vi "Print Footprint v8.1 add to 48 cases.vi"() -> ()   [LabVIEW 2018]
panel:
  in  "Manual Input":string
  out "error out 2":errorcluster
  out "error out":errorcluster
  out "Ring Text":string
  in  "Enter time limit":dbl=10.0
  out "Role":i32[][](array[numeric])=[[1, 0], [3, 0], [10, 0], [18, 0]]
  in  "Manual Input":i32[][](array[numeric])=[[1, 0], [3, 0], [5, 0], [7, 0], [12, 0], [13, 0], [17, 0], [20, 1]]
  out "Numeric 4":i32=7
  out "element":i32=6
  out "Match":u16(ring)=18 items=["0", "1", "2"]
  in  "Select Role":u16(ring)=18 items=["Thyroiditis"=48, "Kidney disease"=47, "Prinzmetal angina"=46, "Gallstones"=45, "Appendicitis"=44, "Heart valve problem"=43, "Enlarged heart"=42, "Staff 20"=41, "Doctor 18"=40, "Doctor 17"=39, "Doctor 16"=38, "Doctor 15"=37, "Doctor 14"=36, "Doctor 13"=35, "Doctor 12"=34, "Nurse 11"=33, "Doctor 10"=32, "Staff 9"=31, "Doctor 8"=30, "Nurse 7"=29, "Doctor 6"=28, "Doctor 5"=27, "Doctor 4"=26, "Doctor 3"=25, "Nurse 1"=24, "Manual Input"=0, "Common cold"=1, "Skin rash"=2, "Anemia"=3, "High blood pressure"=4, "Flu"=5, "Laryngitis"=6, "Strep throat"=7, "Sinus disease"=8, "Sprained wrist"=9, "Sprained ankle"=10, "Allergy"=11, "Lung disease"=12, "Intoxication"=13, "Pneumonia"=14, "Tuberculosis"=15, "Fractured nose"=16, "Fractured rib"=17, "Arrhythmia"=18, "Atherosclerosis"=19, "Anxiety"=20, "Insomnia"=21, "Paranoia"=22, "Diarrhea"=23]
  in  "stop":bool
  in  "Start":bool
  out "Syntetic":i32[][](array[numeric])=[[2, 1], [2, 1], [1, 0], [2, 1], [3, 0], [10, 0], [18, 0]]
  in  "Resting Room #":dbl=20.0
  in  "Toilet Room #":dbl=2.0
  in  "Resting limit":dbl
  in  "Toilet limit":dbl=6.0
  in  "Run for":i32=100
  in  "Enter Rnd Lmt":dbl=2.0
  out "offset past number":i32
  out "for time":i32=2
  out "time":dbl=13.0
  out "at nroom":i32=17
  out "Numeric 3":i32=2
  out "x-1":i32=2
  out "Numeric":i32=13
  out "x+y":dbl
  out "x+1":i32=6
  out "path":path=path "C:/Users/synti/OneDrive/Desktop/NI/new/100.png"
  out "Rec Frame":i32=100
  in  "Record?":bool=TRUE
  out "read":picture
  in  "Entering time":dbl
  out "Footprint":picture
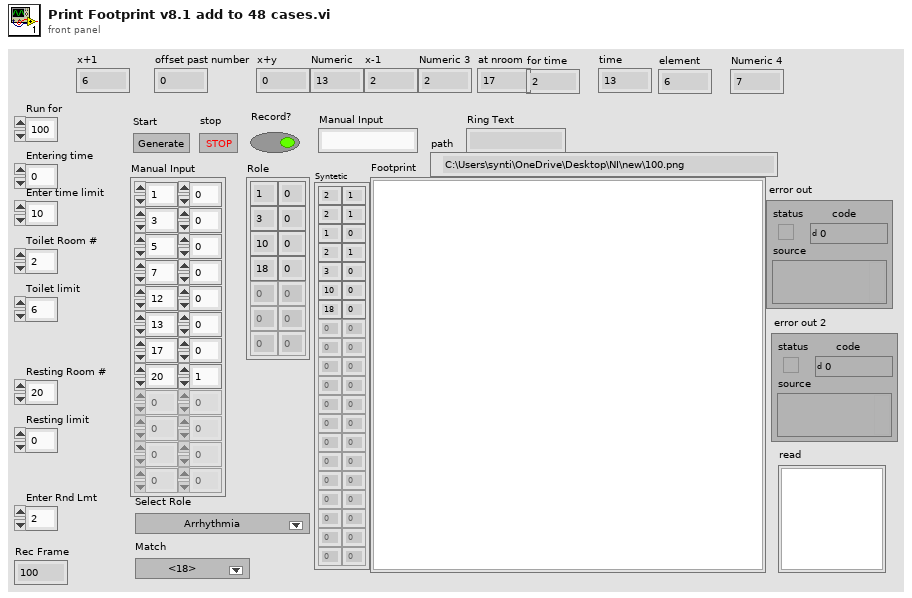
[diagram p1: front panel]
types:
  T1 = typedef "imagedata.ctl" = cluster{"image type":i32, "image depth":i32, "image":u8[], "mask":u8[], "colors":u32[], "Rectangle":cluster{"left":i16, "top":i16, "right":i16, "bottom":i16}}
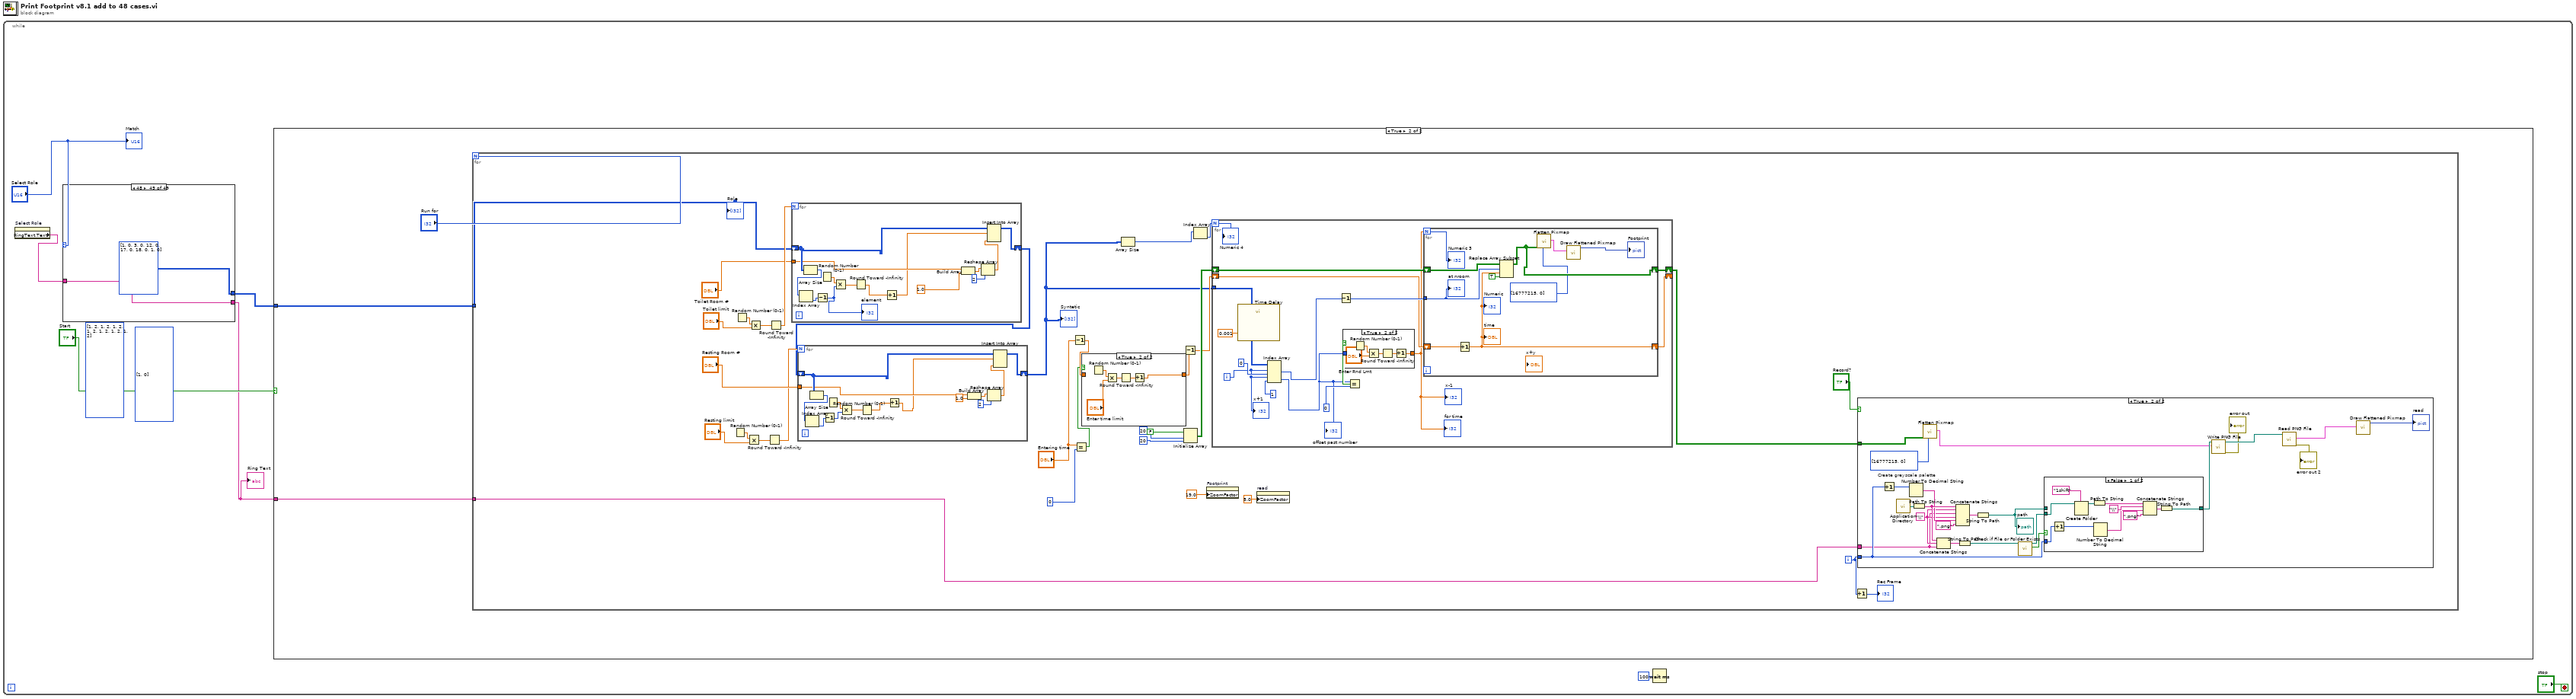
[diagram p0: block diagram]
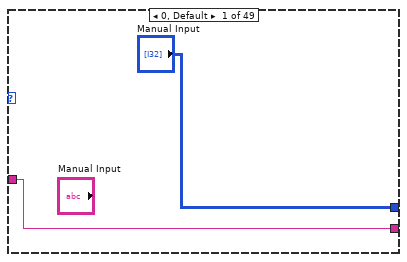
[diagram p2: hidden frame]
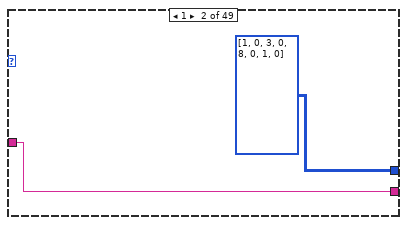
[diagram p3: hidden frame]
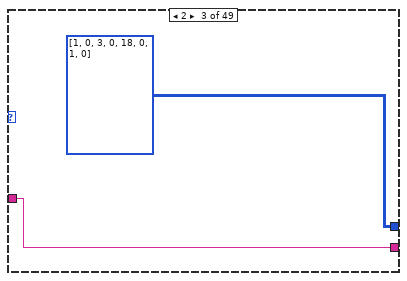
[diagram p4: hidden frame]
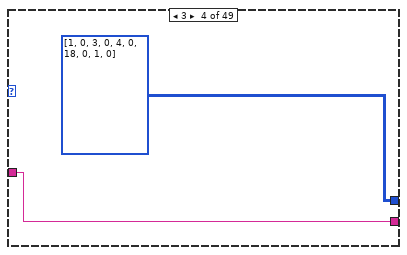
[diagram p5: hidden frame]
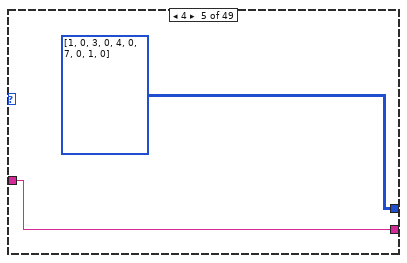
[diagram p6: hidden frame]
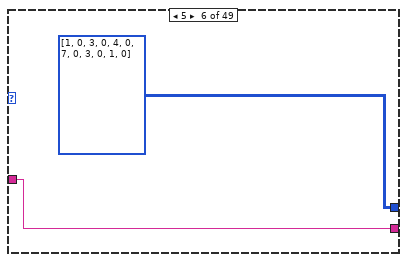
[diagram p7: hidden frame]
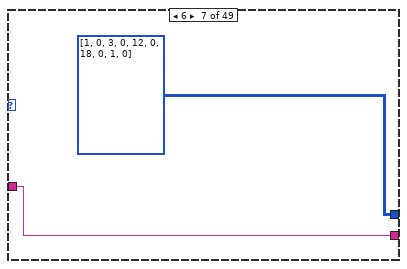
[diagram p8: hidden frame]
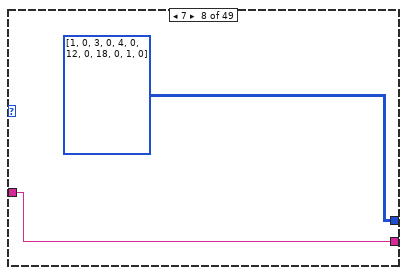
[diagram p9: hidden frame]
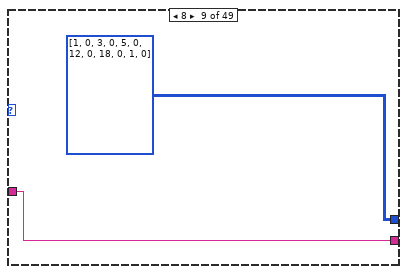
[diagram p10: hidden frame]
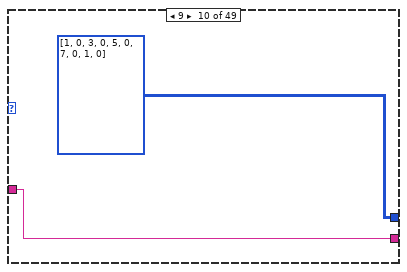
[diagram p11: hidden frame]
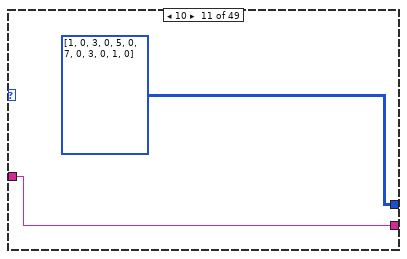
[diagram p12: hidden frame]
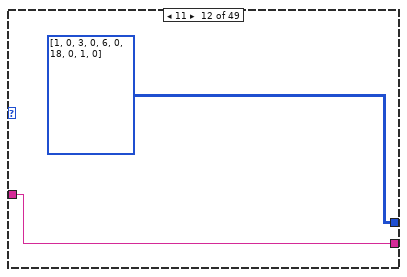
[diagram p13: hidden frame]
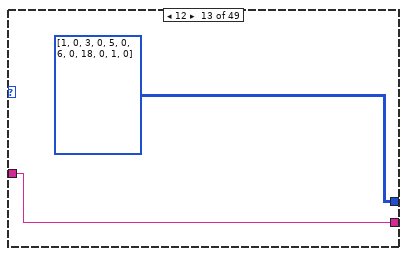
[diagram p14: hidden frame]
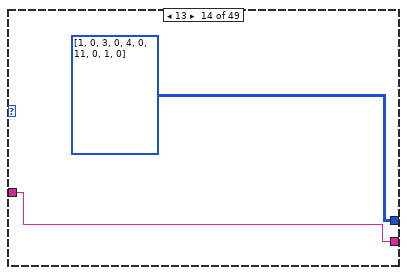
[diagram p15: hidden frame]
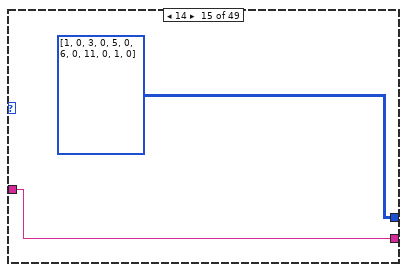
[diagram p16: hidden frame]
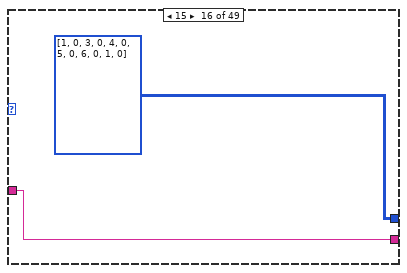
[diagram p17: hidden frame]
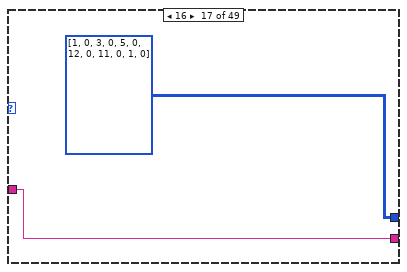
[diagram p18: hidden frame]
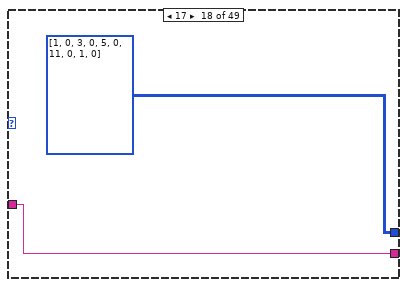
[diagram p19: hidden frame]
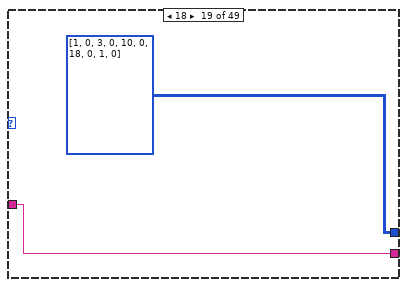
[diagram p20: hidden frame]
diagram:
  n1 = while {
    stop <- "stop" stop-if-true
    (unwired) i32[][] [[1, 0]] ("number 2")
    (unwired) i32[][] [[1, 2], [1, 2], [1, 2], [1, 2], [1, 2], [1, 2], [1, 2]] ("number 2")
    n2 = property on="Select Role" class="Ring (strict)"() -> ("RingText.Text"=w2:string)  [unwired: 2 in, 2 out]
    n3 = case shown="48" "Select Role" {
      tunnel: ["Manual Input" i32[][] [[1, 0], [3, 0], [8, 0], [1, 0]] ("number 2") i32[][] [[1, 0], [3, 0], [18, 0], [1, 0]] ("number 2") i32[][] [[1, 0], [3, 0], [4, 0], [18, 0], [1, 0]] ("number 2") i32[][] [[1, 0], [3, 0], [4, 0], [7, 0], [1, 0]] ("number 2") i32[][] [[1, 0], [3, 0], [4, 0], [7, 0], [3, 0], [1, 0]] ("number 2") i32[][] [[1, 0], [3, 0], [12, 0], [18, 0], [1, 0]] ("number 2") i32[][] [[1, 0], [3, 0], [4, 0], [12, 0], [18, 0], [1, 0]] ("number 2") i32[][] [[1, 0], [3, 0], [5, 0], [12, 0], [18, 0], [1, 0]] ("number 2") i32[][] [[1, 0], [3, 0], [5, 0], [7, 0], [1, 0]] ("number 2") i32[][] [[1, 0], [3, 0], [5, 0], [7, 0], [3, 0], [1, 0]] ("number 2") i32[][] [[1, 0], [3, 0], [6, 0], [18, 0], [1, 0]] ("number 2") i32[][] [[1, 0], [3, 0], [5, 0], [6, 0], [18, 0], [1, 0]] ("number 2") i32[][] [[1, 0], [3, 0], [4, 0], [11, 0], [1, 0]] ("number 2") i32[][] [[1, 0], [3, 0], [5, 0], [6, 0], [11, 0], [1, 0]] ("number 2") i32[][] [[1, 0], [3, 0], [4, 0], [5, 0], [6, 0], [1, 0]] ("number 2") i32[][] [[1, 0], [3, 0], [5, 0], [12, 0], [11, 0], [1, 0]] ("number 2") i32[][] [[1, 0], [3, 0], [5, 0], [11, 0], [1, 0]] ("number 2") i32[][] [[1, 0], [3, 0], [10, 0], [18, 0], [1, 0]] ("number 2") i32[][] [[1, 0], [3, 0], [5, 0], [10, 0], [18, 0], [1, 0]] ("number 2") i32[][] [[1, 0], [3, 0], [8, 0], [18, 0], [1, 0]] ("number 2") i32[][] [[1, 0], [3, 0], [8, 0], [11, 0], [1, 0]] ("number 2") i32[][] [[1, 0], [3, 0], [8, 0], [18, 0], [3, 0], [1, 0]] ("number 2") i32[][] [[1, 0], [3, 0], [13, 0], [18, 0], [1, 0]] ("number 2") i32[][] [[1, 2], [1, 2], [1, 2], [1, 2], [1, 2], [1, 2], [1, 2], [1, 2]] ("number 2") i32[][] [[3, 2], [3, 2], [3, 2], [3, 2], [3, 2], [3, 2], [3, 2]] ("number 2") i32[][] [[4, 2], [4, 2], [4, 2], [4, 2], [4, 2], [4, 2], [4, 2]] ("number 2") i32[][] [[5, 2], [5, 2], [5, 2], [5, 2], [5, 2], [5, 2], [5, 2]] ("number 2") i32[][] [[6, 2], [6, 2], [6, 2], [6, 2], [6, 2], [6, 2], [6, 2]] ("number 2") i32[][] [[7, 2], [7, 2], [7, 2], [7, 2], [7, 2], [7, 2], [7, 2]] ("number 2") i32[][] [[8, 2], [8, 2], [8, 2], [8, 2], [8, 2], [8, 2], [8, 2]] ("number 2") i32[][] [[9, 2], [9, 2], [9, 2], [9, 2], [9, 2], [9, 2], [9, 2]] ("number 2") i32[][] [[10, 2], [10, 2], [10, 2], [10, 2], [10, 2], [10, 2], [10, 2]] ("number 2") i32[][] [[11, 2], [11, 2], [11, 2], [11, 2], [11, 2], [11, 2], [11, 2]] ("number 2") i32[][] [[12, 2], [12, 2], [12, 2], [12, 2], [12, 2], [12, 2], [12, 2]] ("number 2") i32[][] [[13, 2], [13, 2], [13, 2], [13, 2], [13, 2], [13, 2], [13, 2]] ("number 2") i32[][] [[14, 2], [14, 2], [14, 2], [14, 2], [14, 2], [14, 2], [14, 2]] ("number 2") i32[][] [[15, 2], [15, 2], [15, 2], [15, 2], [15, 2], [15, 2], [15, 2]] ("number 2") i32[][] [[16, 2], [16, 2], [16, 2], [16, 2], [16, 2], [16, 2], [16, 2]] ("number 2") i32[][] [[17, 2], [17, 2], [17, 2], [17, 2], [17, 2], [17, 2], [17, 2]] ("number 2") i32[][] [[18, 2], [18, 2], [18, 2], [18, 2], [18, 2], [18, 2], [18, 2]] ("number 2") i32[][] [[20, 2], [20, 2], [20, 2], [20, 2], [20, 2], [20, 2], [20, 2]] ("number 2") i32[][] [[1, 0], [3, 0], [5, 0], [10, 0], [16, 0], [3, 0], [1, 0]] ("number 2") i32[][] [[1, 0], [3, 0], [5, 0], [10, 0], [16, 0], [1, 0]] ("number 2") i32[][] [[1, 0], [3, 0], [13, 0], [16, 0], [11, 0], [1, 0]] ("number 2") i32[][] [[1, 0], [3, 0], [4, 0], [13, 0], [14, 0], [16, 0], [1, 0]] ("number 2") i32[][] [[1, 0], [3, 0], [10, 0], [14, 0], [18, 0], [1, 0]] ("number 2") i32[][] [[1, 0], [3, 0], [17, 0], [13, 0], [7, 0], [1, 0]] ("number 2") i32[][] [[1, 0], [3, 0], [12, 0], [17, 0], [18, 0], [1, 0]] ("number 2")] -> w4
      tunnel: w2 -> [w8 w10 w12 w14 w16 w18 w20 w22 w24 w26 w28 w30 w32 w34 w36 w38 w40 w42 w44 w46 w48 w50 w52 w54 w56 w58 w60 w62 w64 w66 w68 w70 w72 w74 w76 w78 w80 w82 w84 w86 w88 w90 w92 w94 w96 w98 w100 w102 w104]
      tunnel: [w8 w10 w12 w14 w16 w18 w20 w22 w24 w26 w28 w30 w32 w34 w36 w38 w40 w42 w44 w46 w48 w50 w52 w54 w56 w58 w60 w62 w64 w66 w68 w70 w72 w74 w76 w78 w80 w82 w84 w86 w88 w90 w92 w94 w96 w98 w100 w102 w104] -> w1
      frame 0, Default {
      }
      frame 1 {
      }
      frame 2 {
      }
      frame 3 {
      }
      frame 4 {
      }
      frame 5 {
      }
      frame 6 {
      }
      frame 7 {
      }
      frame 8 {
      }
      frame 9 {
      }
      frame 10 {
      }
      frame 11 {
      }
      frame 12 {
      }
      frame 13 {
      }
      frame 14 {
      }
      frame 15 {
      }
      frame 16 {
      }
      frame 17 {
      }
      frame 18 {
      }
      frame 19 {
      }
      frame 20 {
      }
      frame 21 {
      }
      frame 22 {
      }
      frame 23 {
      }
      frame 24 {
      }
      frame 25 {
      }
      frame 26 {
      }
      frame 27 {
      }
      frame 28 {
      }
      frame 29 {
      }
      frame 30 {
      }
      frame 31 {
      }
      frame 32 {
      }
      frame 33 {
      }
      frame 34 {
      }
      frame 35 {
      }
      frame 36 {
      }
      frame 37 {
      }
      frame 38 {
      }
      frame 39 {
      }
      frame 40 {
      }
      frame 41 {
      }
      frame 42 {
      }
      frame 43 {
      }
      frame 44 {
      }
      frame 45 {
      }
      frame 46 {
      }
      frame 47 {
      }
      frame 48 {
      }
    }
    "Ring Text" <- w1
    n4 = case shown="True" "Start" {
      tunnel: w4 -> [_ w107]
      tunnel: w1 -> [_ w106]
      frame False {
      }
      frame True {
        n5 = for {
          N: "Run for" -> [_]
          tunnel: w107 -> [w116]
          tunnel: w106 -> [w109]
          i -> [w137]
          n6 = Random Number (0-1)() -> (number: 0 to 1=w128:dbl)
          n7 = Random Number (0-1)() -> (number: 0 to 1=w130:dbl)
          n8 = Multiply(x=w128, y="Resting limit") -> (x*y=w127:dbl)
          n9 = Multiply(x=w130, y="Toilet limit") -> (x*y=w129:dbl)
          n10 = Round Toward -Infinity(1:w127) -> (0:w122:dbl)
          n11 = Round Toward -Infinity(1:w129) -> (0:w126:dbl)
          n12 = for {
            N: w126 -> [_]
            shift-right: [w166] -> w119
            shift-left: w116 -> [w172]
            tunnel: "Toilet Room #" -> [w170]
            n13 = Array Size(array=w172) -> (size(s)=w171:i32[])
            n14 = Index Array(array=w171) -> (element=w162:i32)  [unwired: 1 in]
            n15 = Decrement(x=w162) -> (x-1=w161:i32)
            "element" <- w161
            n16 = Random Number (0-1)() -> (number: 0 to 1=w174:dbl)
            n17 = Multiply(x=w174, y=w161) -> (x*y=w173:dbl)
            n18 = Round Toward -Infinity(1:w173) -> (0:w164:dbl)
            n19 = Increment(x=w164) -> (x+1=w163:dbl)
            n20 = Build Array(w170, 1.0 ("y")) -> (w169:dbl[])
            n21 = Reshape Array(w169, 2 ("dimension size")) -> (w167:dbl[])
            n22 = Insert Into Array(array=w172, index (row)=w163, new element=w167) -> (w166:i32[][])  [unwired: 1 in]
          }
          n23 = for {
            N: w122 -> [_]
            shift-right: [w156] -> w117
            shift-left: w119 -> [w158]
            tunnel: "Resting Room #" -> [w155]
            n24 = Array Size(array=w158) -> (size(s)=w157:i32[])
            n25 = Index Array(array=w157) -> (element=w148:i32)  [unwired: 1 in]
            n26 = Decrement(x=w148) -> (x-1=w147:i32)
            n27 = Random Number (0-1)() -> (number: 0 to 1=w160:dbl)
            n28 = Multiply(x=w160, y=w147) -> (x*y=w159:dbl)
            n29 = Round Toward -Infinity(1:w159) -> (0:w150:dbl)
            n30 = Increment(x=w150) -> (x+1=w149:dbl)
            n31 = Build Array(w155, 1.0 ("element")) -> (w154:dbl[])
            n32 = Reshape Array(w154, 2 ("dimension size")) -> (w152:dbl[])
            n33 = Insert Into Array(array=w158, index (row)=w149, new element=w152) -> (w156:i32[][])  [unwired: 1 in]
          }
          "Syntetic" <- w117
          n34 = Decrement(x="Entering time") -> (x-1=w112:dbl)
          n35 = Equal?(x="Entering time", y=0) -> (x = y?=w110:bool)
          n36 = case shown="True" w110 {
            tunnel: w112 -> [w141 _]
            tunnel: [w141 w142] -> w111
            frame False {
            }
            frame True {
              n37 = Random Number (0-1)() -> (number: 0 to 1=w146:dbl)
              n38 = Multiply(x=w146, y="Enter time limit") -> (x*y=w144:dbl)
              n39 = Round Toward -Infinity(1:w144) -> (0:w145:dbl)
              n40 = Increment(x=w145) -> (x+1=w142:dbl)
            }
          }
          n41 = Array Size(array=w117) -> (size(s)=w131:i32[])
          n42 = Decrement(x=w111) -> (x-1=w132:dbl)
          n43 = Initialize Array(FALSE, 20 ("dimension size"), 20 ("dimension size")) -> (w133:bool[][])
          n44 = Index Array(array=w131) -> (element=w136:i32)  [unwired: 1 in]
          n45 = property on="Footprint" class="Pict"("ZoomFactor"=sgl 19.0 ("Zoom Factor")) -> ()  [unwired: 2 in, 2 out]
          n46 = for {
            N: w136 -> [w210]
            tunnel: w117 -> [w225]
            shift-right: [w220] -> w118
            shift-left: w133 -> [w221]
            shift-right: [w219] -> _
            shift-left: w132 -> [w217]
            i -> [w213]
            n47 = call "Time Delay"("Delay Time (s)"=0.001) -> ()  [unwired: 10 in, 1 out]
            n48 = Index Array(array=w225, index (row) #1=w213, index (col) #1=0 ("disabled index (col)"), index (row) #2=w213, index (col) #2=1 ("disabled index (col)")) -> (element #1=w212:i32, element #2=w211:i32)
            "offset past number" <- w211
            n49 = Decrement(x=w212) -> (x-1=w218:i32)
            n50 = Equal?(x=w211, y=0) -> (x = y?=w216:bool)
            n51 = case shown="True" w216 {
              tunnel: w211 -> [w226 _]
              tunnel: [w226 w228] -> w214
              frame False {
              }
              frame True {
                n52 = Random Number (0-1)() -> (number: 0 to 1=w231:dbl)
                n53 = Multiply(x=w231, y="Enter Rnd Lmt") -> (x*y=w229:dbl)
                n54 = Round Toward -Infinity(1:w229) -> (0:w230:dbl)
                n55 = Increment(x=w230) -> (x+1=w228:dbl)
              }
            }
            "x-1" <- w214
            "for time" <- w214
            n56 = for {
              N: w214 -> [w238]
              tunnel: w218 -> [w235]
              shift-right: [w236] -> w219
              shift-left: w217 -> [w237]
              shift-right: [w233] -> w220
              shift-left: w221 -> [w241]
              n57 = Increment(x=w237) -> (x+1=w236:dbl)
              "Numeric" <- w236
              "time" <- w236
              n58 = Replace Array Subset(array=w241, new element=TRUE ("new element/subarray"), index (row)=w235, index (col)=w236) -> (w233:bool[][])
              n59 = call <vilib>:"Flatten Pixmap.vi"("colors"=u32[] [16777215, 0], "1-bit pixmap"=w233) -> ("image data"=w240:T1)  [unwired: 9 in]
              n60 = call <vilib>:"Draw Flattened Pixmap.vi"("image data"=w240) -> ("new picture"=→"Footprint":picture)  [unwired: 8 in]
              "Numeric 3" <- w238
              "at nroom" <- w235
            }
            "x+1" <- w213
            "Numeric 4" <- w210
          }
          n61 = property on="read" class="Pict"("ZoomFactor"=sgl 5.0 ("Zoom Factor")) -> ()  [unwired: 2 in, 2 out]
          n62 = Increment(x=w137) -> (x+1=→"Rec Frame":i32)
          n63 = case shown="True" "Record?" {
            tunnel: w137 -> [_ w184]
            tunnel: w118 -> [_ w180]
            tunnel: w109 -> [_ w177]
            frame False {
            }
            frame True {
              w181 = "\\" ("string")
              # "Create greyscale palette"
              n64 = Increment(x=w184) -> (x+1=w193:i32)
              n65 = call <vilib>:"Application Directory.vi"() -> ("Application Directory"=w191:path)
              n66 = Number To Decimal String(number=w193) -> (decimal integer string=w182:string)  [unwired: 1 in]
              n67 = Path To String(path=w191) -> (string=w190:string)
              n68 = call <vilib>:"Flatten Pixmap.vi"("colors"=u32[] [16777215, 0], "1-bit pixmap"=w180) -> ("image data"=w179:T1)  [unwired: 9 in]
              n69 = Concatenate Strings(w190, w181, w177) -> (w188:string)
              n70 = Concatenate Strings(w190, w181, w177, w181, w182, ".png" ("string")) -> (w197:string)
              n71 = String To Path(string=w188) -> (path=w189:path)
              n72 = String To Path(string=w197) -> (path=w186:path)
              "path" <- w186
              n73 = call <vilib>:"Check if File or Folder Exists.vi"("path"=w189) -> ("file or folder exists?"=w192:bool, "dup path"=w187:path)  [unwired: 8 in, 1 out]
              n74 = case shown="False" w192 {
                tunnel: w187 -> [w208 _]
                tunnel: w186 -> [_ w209]
                tunnel: [w200 w209] -> w185
                tunnel: w184 -> [w203 _]
                frame False {
                  n75 = Increment(x=w203) -> (x+1=w205:i32)
                  n76 = Create Folder(prompt (Create Folder)="1shift", path (use dialog)=w208) -> (created path=w202:path)  [unwired: 1 in, 2 out]
                  n77 = Path To String(path=w202) -> (string=w201:string)
                  n78 = Number To Decimal String(number=w205) -> (decimal integer string=w199:string)  [unwired: 1 in]
                  n79 = Concatenate Strings(w201, "\\" ("string"), w199, ".png" ("string")) -> (w206:string)
                  n80 = String To Path(string=w206) -> (path=w200:path)
                }
                frame True {
                }
              }
              n81 = call <vilib>:"Write PNG File.vi"("image data"=w179, "path to PNG file"=w185) -> ("error out"=→"error out":errorcluster, "path"=w194:path)  [unwired: 8 in]
              n82 = call <vilib>:"Read PNG File.vi"("path to PNG file"=w194) -> ("error out"=→"error out 2":errorcluster, "image data"=w196:T1)  [unwired: 8 in, 1 out]
              n83 = call <vilib>:"Draw Flattened Pixmap.vi"("image data"=w196) -> ("new picture"=→"read":picture)  [unwired: 8 in]
            }
          }
          "Role" <- w116
        }
      }
    }
    n84 = Wait (ms)(milliseconds to wait=u32 100) -> ()  [unwired: 1 out]
    "Match" <- "Select Role"
  }
